vi "GUI_laptop v11i.vi"() -> ()   [LabVIEW 2019]
uses:
  <vilib>/Math Plots/3D Math Plots/3D Scatter/3D Scatter XCtrl/3D Scatter.xctl
  <vilib>/Platform/TimedLoop/XDataNode/timing_clust.ctl
  <vilib>/Platform/TimedLoop/XDataNode/nitl_modes.ctl
  <vilib>/Platform/TimedLoop/XDataNode/wakeup.ctl
  <vilib>/Analysis/_algsub.llb/Real Vector Norm.vi
  <vilib>/Instr/_visa.llb/VISA Configure Serial Port (Instr).vi
  <vilib>/Utility/file.llb/Write Delimited Spreadsheet (DBL).vi
  <vilib>/addons/System Identification/Data Preprocess.llb/SI Lowpass Filter (MISO Array).vi
  <vilib>/Math Plots/3D Math Plots/3D Scatter/3D Scatter Datatype/Public/Plot Helper (Vector).vi
  <vilib>/platform/TimedLoop/XDataNode/XDataNode.xnode
  <vilib>/Platform/TimedLoop/XDataNode/XDNodeRunTimeDep.lvlib
  <vilib>/Analysis/NI_AALPro.lvlib
  <vilib>/Math Plots/3D Math Plots/3D Scatter/3D Scatter Datatype/3D Scatter Datatype.lvclass
  <vilib>/addons/System Identification/NI_SysID.lvlib
panel:
  out "Period":i64
  out "Actual End [i-1]":i64
  out "Expected End [i-1]":i64
  out "Finished Late? [i-1] 2":bool
  in  "l3_init":dbl=2.0
  in  "Motion scale L3 outside rcm":dbl=2.0
  in  "L5 Deadzone":dbl
  in  "Sample rate":u32=500
  in  "Cutoff Frequency":dbl=10.0
  in  "Motion scale L1 L2":dbl=10.0
  in  "Motion scale L3":dbl=2.0
  in  "Save Path 4":path=path "C:/Users/jimmy/Documents/GitHub/Arduino-LabVIEW/zhantao/read_data_abs_filtered.csv"
  in  "Save Path 3":path=path "C:/Users/jimmy/Documents/GitHub/Arduino-LabVIEW/zhantao/read_data_abs_sending.csv"
  out "stimulus signals out":dbl[][](array[numeric]) format="%.2f"
  in  "L5 Offset":dbl
  in  "L5 Scale":dbl=1.0
  in  "Motion Scale L4":dbl=30.0
  out "spreadsheet string":string
  in  "Save Path 2":path=path "C:/Users/jimmy/Documents/GitHub/Arduino-LabVIEW/zhantao/read_data_delt.csv"
  out "send values":dbl[](array[numeric])
  out "Robot Feedback (l1 l2 l3 l4)":dbl[](array[numeric])
  in  "UDP Send":bool
  in  "UDP Recv":bool
  in  "L5 bound":dbl=1000.0
  in  "L4 bound (deg)":dbl=1000.0
  in  "L3 bound (mm)":dbl=1000.0
  in  "L2 bound (deg)":dbl=1000.0
  in  "L1 bound (deg)":dbl=1000.0
  in  "Joystick Type":dbl(ring)=1.0 items=["Rigid Joystick", "Free Joystick"]
  out "Finished Late? [i-1]":bool
  in  "Epsilon":dbl=0.2
  out "3D Scatter":refnum<class "3D Plot Datatype.lvclass">[](xcontrol)
  out "Random Point":dbl[](array[numeric])
  out "Virtual Cursor":dbl[](array[numeric])
  out "Iteration Duration":i64
  in  "Num of Points":i32=10
  in  "z bound":dbl=2.0
  in  "y bound":dbl=5.0
  in  "x bound":dbl=5.0
  in  "Stop":bool
  in  "Round Decimals":dbl=2.0 format="%#_15g"
  in  "Save Data":bool
  in  "Save Path":path=path "C:/Users/jimmy/Documents/GitHub/Arduino-LabVIEW/zhantao/read_data_abs.csv"
  in  "x speed":dbl=0.5
  in  "z speed":dbl=0.5
  in  "y speed":dbl=0.5
  out "error out":errorcluster
  in  "baud rate":u32=250000
  in  "VISA resource name":refnum<visa-resource-name>
  # "Joystick Selection"
  # "Plotting"
  # "Data Saving"
  # "Arduino Communication"
  # "Master Slave Communication"
  # "Parameters"
  # "TODO: add a lowpass filter for l5"
  # "TODO: fix the bounds; currently bounds are arbitrary"
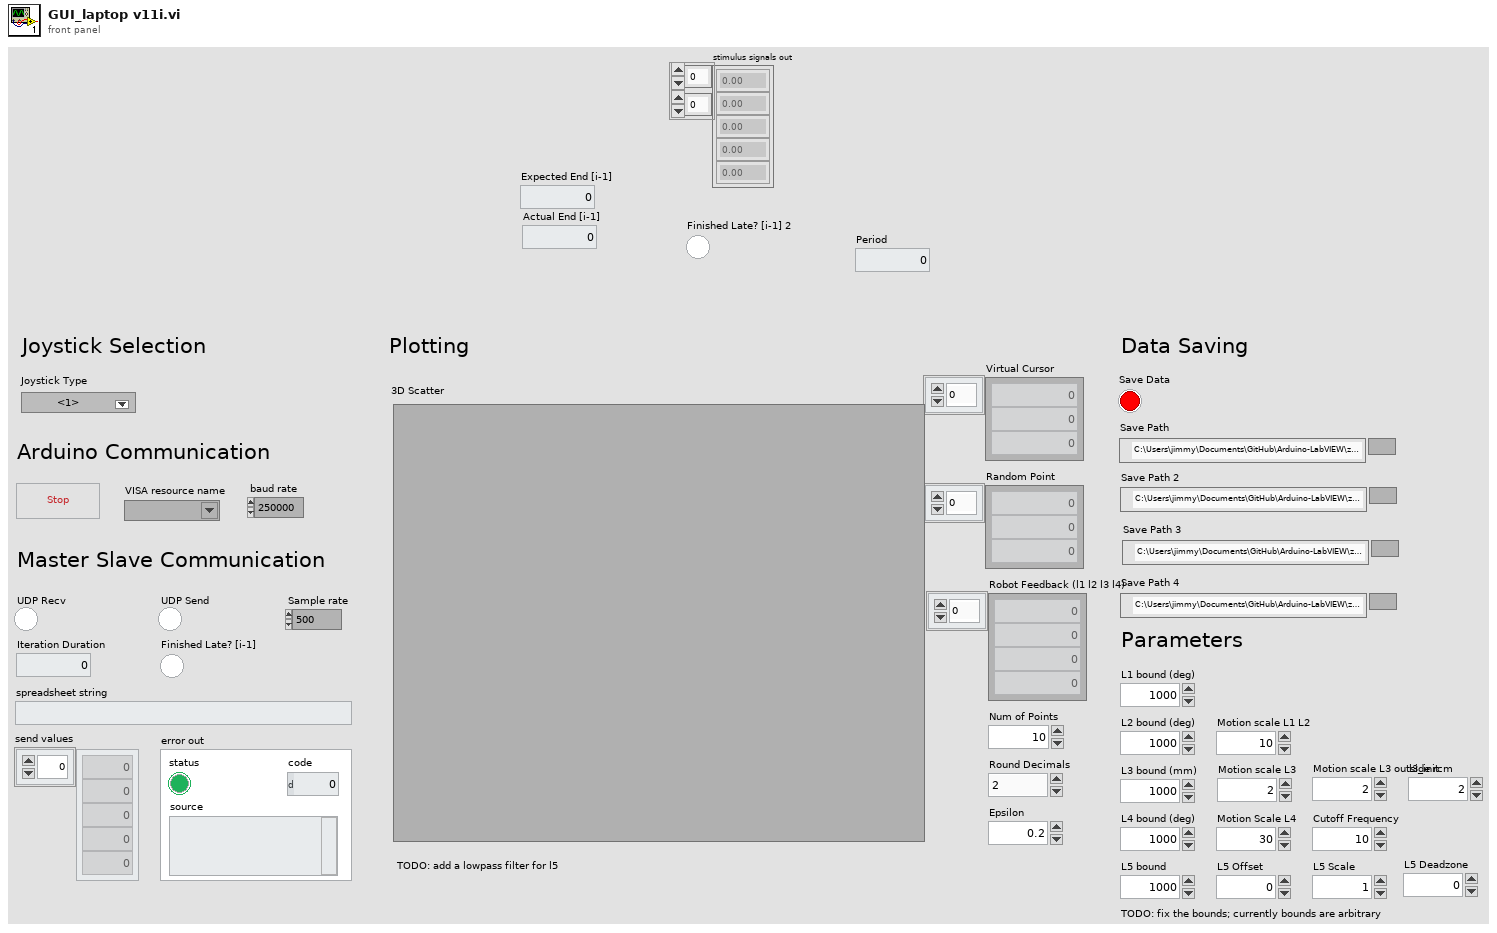
[diagram p1: front panel]
types:
  T1 = typedef "XDNodeRunTimeDep.lvlib/timing_clust.ctl" = cluster{"Expected End [f-1]":u64, "Actual End [f-1]":u64, "Finished Late? [f-1]":bool, "Expected End [i-1]":u64, "Actual End [i-1]":u64, "Finished Late? [i-1]":bool, "Expected Start [i]":u64, "Actual Start [i]":u64, "Expected Start [f]":u64, "Actual Start [f]":u64, "Source Name":string, "Structure Name":string, "Period":i64, "Deadline":i64, "Offset":i64, "Start":i64, "Priority":i32, "Timeout":i32, "Mode":T2, "Wakeup Reason":T3, "Error":errorcluster, "Source Type":string, "Secondary Source Type":string, "Global End Time":u64, "Global Start Time":u64, "Frame Duration":u64, "Iteration Duration":u64, "Assigned CPU":i32, "I/O Scan Engine Mode":u32}
  T2 = typedef "XDNodeRunTimeDep.lvlib/nitl_modes.ctl" = enum32{"No Change", "Process missed periods, maintain original phase", "Discard missed periods, maintain original phase", "Process missed periods, ignore original phase", "Discard missed periods, ignore original phase"}
  T3 = typedef "XDNodeRunTimeDep.lvlib/wakeup.ctl" = enum32{"Normal", "Aborted", "Asynchronous wakeup", "Timing source error", "Timed loop error", "Timeout"}
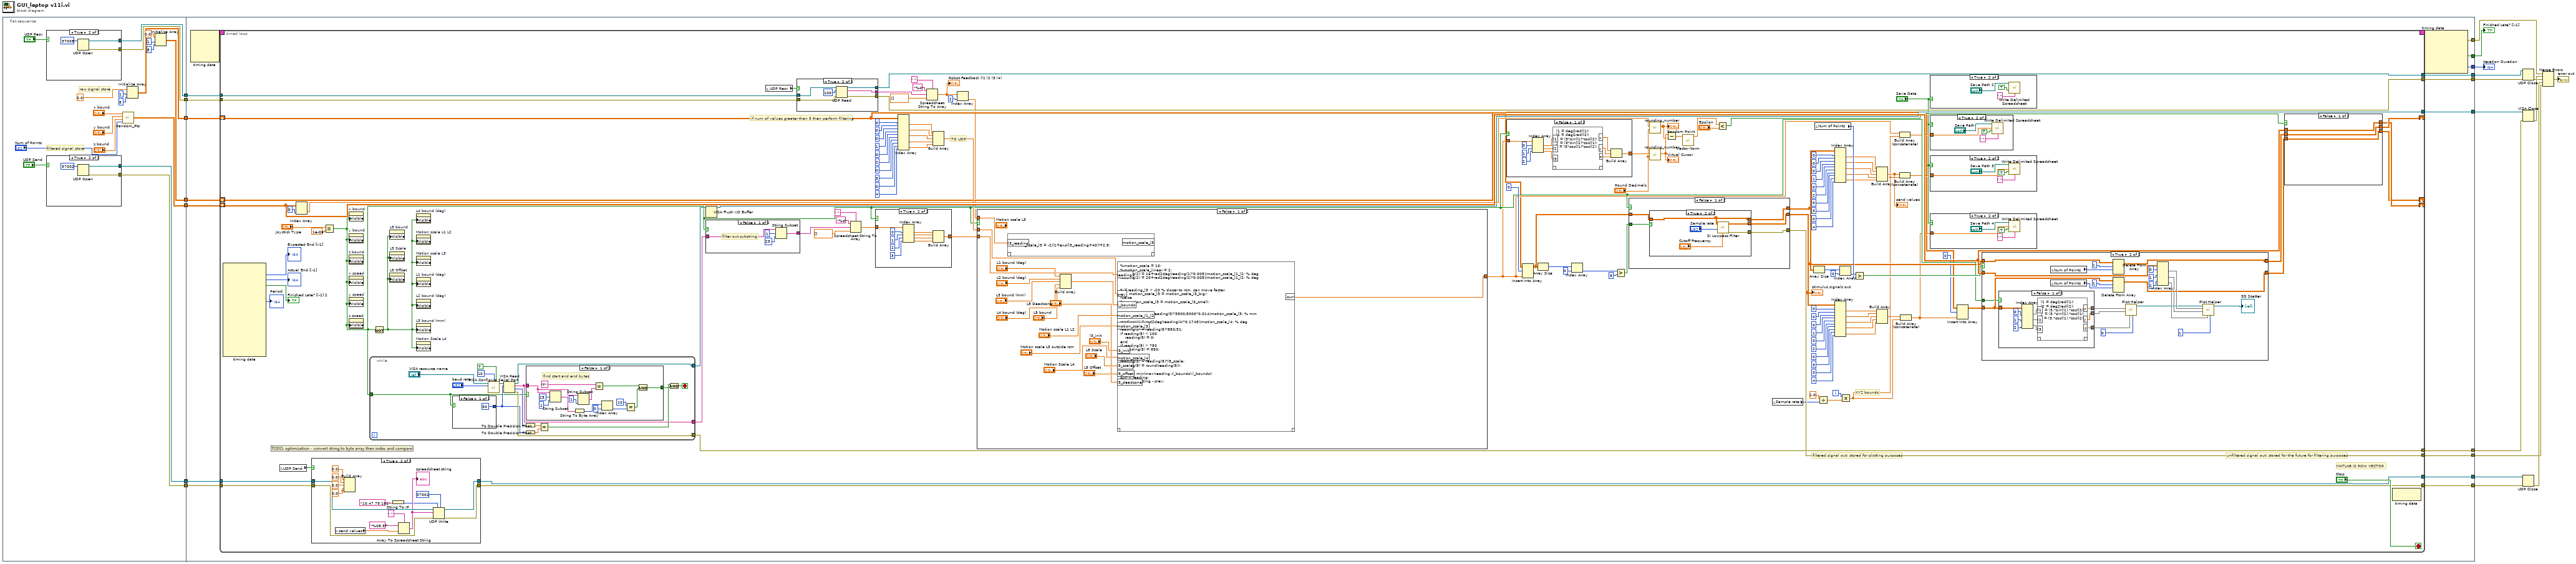
[diagram p0: block diagram]
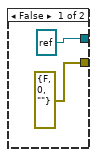
[diagram p2: hidden frame]
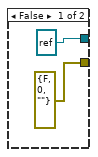
[diagram p3: hidden frame]
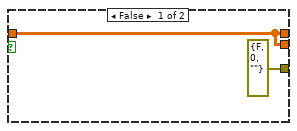
[diagram p6: hidden frame]
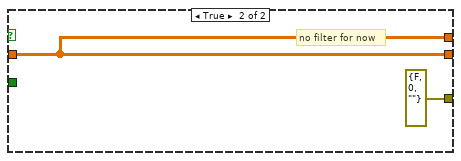
[diagram p7: hidden frame]
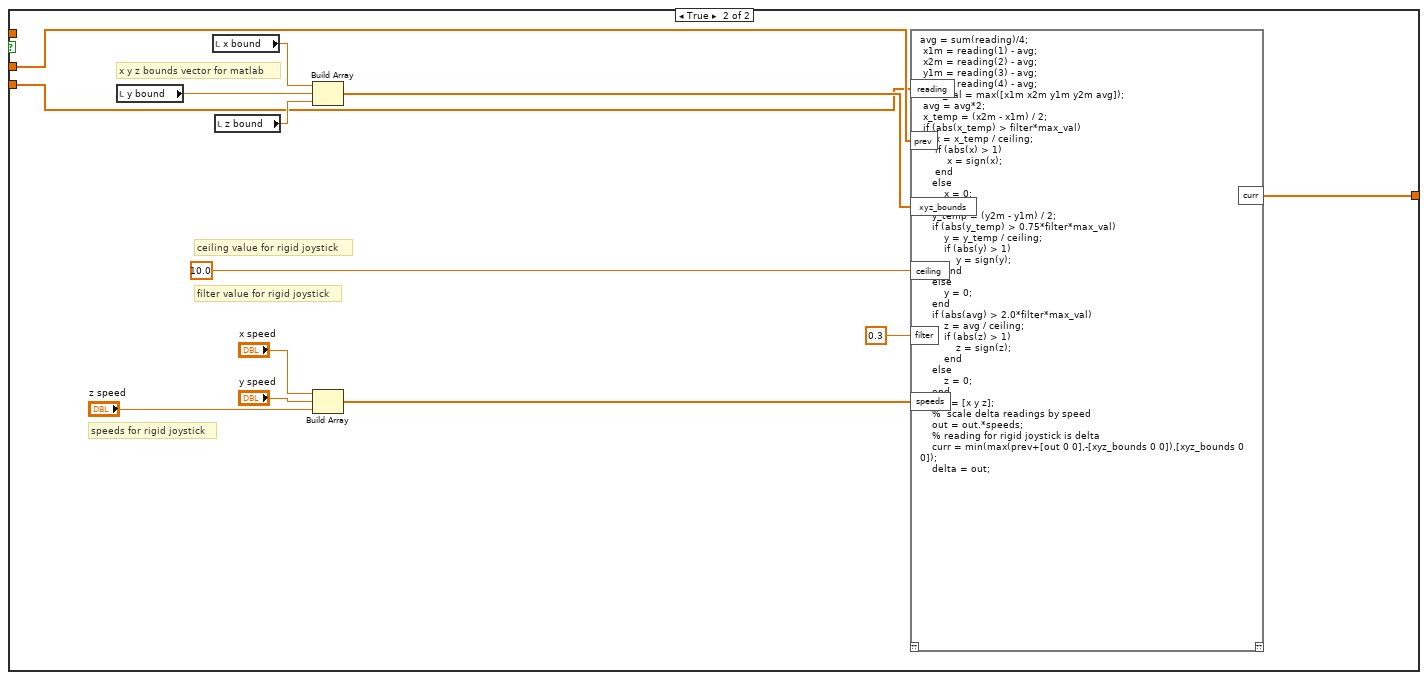
[diagram p8: hidden frame]
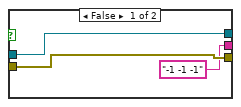
[diagram p11: hidden frame]
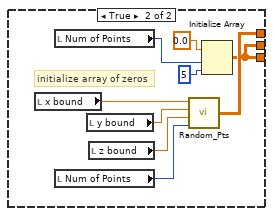
[diagram p13: hidden frame]
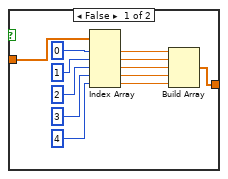
[diagram p15: hidden frame]
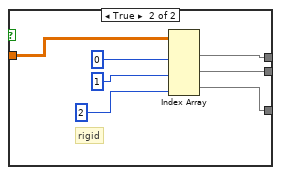
[diagram p18: hidden frame]
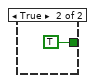
[diagram p19: hidden frame]
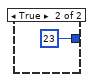
[diagram p20: hidden frame]
diagram:
  n1 = flat-sequence {
    tunnel: [w32] -> w18
    tunnel: [w36] -> w17
    tunnel: [w31] -> w16
    tunnel: [w30] -> w15
    tunnel: [w27] -> w14
    tunnel: [w26] -> w13
    tunnel: [w22] -> w2
    tunnel: [w67] -> w21
    tunnel: [w66] -> w20
    tunnel: [w64] -> w12
    tunnel: [w62] -> w19
    tunnel: w18 -> [w65]
    tunnel: w17 -> [w63]
    tunnel: w16 -> [w61]
    tunnel: w15 -> [w60]
    tunnel: w14 -> [w59]
    tunnel: w13 -> [w58]
    tunnel: [w57] -> w6
    tunnel: [w56] -> w11
    tunnel: [w55] -> w5
    tunnel: [w54] -> w4
    tunnel: [w53] -> w3
    tunnel: w2 -> [w52]
    tunnel: [w51] -> w1
    frame #0 {
      # "filtered signal store"
      # "raw signal store"
      n2 = case shown="True" "UDP Recv" {
        tunnel: [refnum<k16> refnum ("port") w49] -> w30
        tunnel: [errorcluster {"status"=FALSE, "code"=0, "source"=""} ("error out") w48] -> w27
        frame False {
        }
        frame True {
          n3 = UDP Open(11:u16 37008 ("port")) -> (port=w49:refnum<k16>, 0:w48:errorcluster)  [unwired: 4 in, 1 out]
        }
      }
      n4 = case shown="True" "UDP Send" {
        tunnel: [refnum<k16> refnum ("port") w44] -> w31
        tunnel: [errorcluster {"status"=FALSE, "code"=0, "source"=""} ("error out") w43] -> w26
        frame False {
        }
        frame True {
          n5 = UDP Open(11:u16 37002 ("port")) -> (port=w44:refnum<k16>, 0:w43:errorcluster)  [unwired: 4 in, 1 out]
        }
      }
      n6 = call "Random_Pts.vi"("Num of Points"="Num of Points", "z bound"="z bound", "y bound"="y bound", "x bound"="x bound") -> ("appended array"=w36:dbl[][])
      n7 = Initialize Array(0.0 ("element"), 1 ("dimension size"), 5 ("dimension size")) -> (w32:dbl[][])
      n8 = Initialize Array(0.0 ("element"), 1 ("dimension size"), 5 ("dimension size")) -> (w22:dbl[][])
    }
    frame #1 {
      n9 = node-c288() -> (w69:T1)  [unwired: 4 in]
      n10 = timed-loop {
        tunnel: [w141] -> w67
        tunnel: [w197] -> w66
        shift-right: [w196] -> _
        shift-left: w65 -> [w95]
        timing: w69 -> [_]
        timing-out: [_] -> w68
        shift-right: [w192] -> _
        shift-left: w63 -> [w193]
        tunnel: w61 -> [w155]
        tunnel: w60 -> [w154]
        tunnel: w59 -> [w152]
        tunnel: w58 -> [w151]
        tunnel: [w150] -> w57
        tunnel: [w149] -> w56
        tunnel: [w148] -> w55
        tunnel: [w147] -> w54
        tunnel: [w130] -> w53
        shift-right: [w86] -> _
        shift-left: w52 -> [w89]
        i -> [w84]
        stop <- "Stop" stop-if-true
        # "unfiltered signal out; stored for the future for filtering purposes"
        # "filtered signal out; stored for plotting purposes"
        # "XYZ bounds"
        # "if num of values greater than 5 then perform filtering"
        # "TO UDP"
        # "MATLAB IS ROW VECTOR"
        n11 = node-c288() -> (→"Expected End [i-1]":i64, →"Actual End [i-1]":i64, →"Finished Late? [i-1] 2":bool, →"Period":i64)  [unwired: 1 in, 12 out]
        n12 = local read "UDP Send"() -> (w79:bool)
        n13 = Index Array(array=w193, index (col)=0 ("index (row)")) -> (element=w164:dbl[])  [unwired: 1 in]
        n14 = case shown="True" w79 {
          tunnel: w155 -> [w254 w270]
          tunnel: w151 -> [w255 w266]
          tunnel: [w255 w262] -> w149
          tunnel: [w254 w261] -> w147
          frame False {
          }
          frame True {
            w260 = 0.0 ("element")
            n15 = local read "send values"() -> (w256:dbl[])
            n16 = Build Array(0.0 ("element"), 0.0 ("element"), 0.0 ("element"), w260, w260) -> ()  [unwired: 1 out]
            n17 = String To IP(1:"10.47.79.181" ("name")) -> (0:w264:u32)
            n18 = Array To Spreadsheet String(delimiter (Tab)=" ", array=w256, 3:"%08.3f" ("format string")) -> (spreadsheet string=w267:string)
            "spreadsheet string" <- w267
            n19 = UDP Write(address=w264, port or service name=u16 37001, connection ID=w270, data in=w267, 8:w266) -> (error out=w262:errorcluster, 3:w261:refnum<k16>)  [unwired: 1 in]
          }
        }
        n20 = Less Or Equal?(x="Joystick Type", y=1e-06) -> (x <= y?=w131:bool)
        n21 = property on="x bound" class="DigNum (strict)"("Visible"=w131) -> ()  [unwired: 2 in, 2 out]
        n22 = property on="y bound" class="DigNum (strict)"("Visible"=w131) -> ()  [unwired: 2 in, 2 out]
        n23 = property on="z bound" class="DigNum (strict)"("Visible"=w131) -> ()  [unwired: 2 in, 2 out]
        n24 = property on="x speed" class="DigNum (strict)"("Visible"=w131) -> ()  [unwired: 2 in, 2 out]
        n25 = property on="y speed" class="DigNum (strict)"("Visible"=w131) -> ()  [unwired: 2 in, 2 out]
        n26 = property on="z speed" class="DigNum (strict)"("Visible"=w131) -> ()  [unwired: 2 in, 2 out]
        n27 = while {
          tunnel: [w377] -> w166
          tunnel: [w390] -> w197
          tunnel: [w384] -> w142
          tunnel: w131 -> [w378]
          stop <- w380 stop-if-true
          n28 = case shown="False" w378 {
            tunnel: [30 u32 23 ("byte count")] -> w383
            frame False {
            }
            frame True {
            }
          }
          n29 = call-poly "VISA Configure Serial Port"("VISA resource name"="VISA resource name", "termination char\n(0xA = '\\n' = LF)"=u8 10 ("termination char\n(0xA = '\\n' = LF)"), "Enable Termination\nChar (T)"=TRUE ("Enable Termination\nChar (T)"), "baud rate (9600)"="baud rate") -> ("VISA resource name out"=w385:refnum<visa-resource-name>)  [unwired: 10 in, 1 out]
          n30 = VISA Read(VISA resource name=w385, byte count=w383) -> (VISA resource name out=w384:refnum<visa-resource-name>, read buffer=w377:string, return count=w392:u32, error out=w390:errorcluster)  [unwired: 1 in]
          n31 = To Double Precision Float(number=w392) -> (double precision float=w391:dbl)
          n32 = To Double Precision Float(number=w383) -> (double precision float=w382:dbl)
          n33 = case shown="False" w378 {
            tunnel: [w399 TRUE] -> w379
            tunnel: w377 -> [w402 _]
            frame False {
              # "find start and end bytes"
              n34 = String Subset(string=w402, offset (0)=29, length (rest)=1) -> (substring=w397:string)
              n35 = String To Byte Array(string=w397) -> (unsigned byte array=w396:u8[])
              n36 = String Subset(string=w402, length (rest)=1) -> (substring=w405:string)  [unwired: 1 in]
              n37 = Equal?(x="T", y=w405) -> (x = y?=w401:bool)
              n38 = Index Array(array=w396, index=0) -> (element=w394:u8)
              n39 = Equal?(x=10, y=w394) -> (x = y?=w400:bool)
              n40 = And(x=w401, y=w400) -> (x .and. y?=w399:bool)
            }
            frame True {
            }
          }
          n41 = Equal?(x=w391, y=w382) -> (x = y?=w381:bool)
          n42 = And(x=w381, y=w379) -> (x .and. y?=w380:bool)
        }
        n43 = Not(x=w131) -> (.not. x?=w93:bool)
        n44 = property on="L5 bound" class="DigNum (strict)"("Visible"=w93) -> ()  [unwired: 2 in, 2 out]
        n45 = property on="L5 Scale" class="DigNum (strict)"("Visible"=w93) -> ()  [unwired: 2 in, 2 out]
        n46 = property on="L5 Offset" class="DigNum (strict)"("Visible"=w93) -> ()  [unwired: 2 in, 2 out]
        n47 = property on="L4 bound (deg)" class="DigNum (strict)"("Visible"=w93) -> ()  [unwired: 2 in, 2 out]
        n48 = property on="Motion scale L1 L2" class="DigNum (strict)"("Visible"=w93) -> ()  [unwired: 2 in, 2 out]
        n49 = property on="Motion scale L3" class="DigNum (strict)"("Visible"=w93) -> ()  [unwired: 2 in, 2 out]
        n50 = property on="L1 bound (deg)" class="DigNum (strict)"("Visible"=w93) -> ()  [unwired: 2 in, 2 out]
        n51 = property on="L2 bound (deg)" class="DigNum (strict)"("Visible"=w93) -> ()  [unwired: 2 in, 2 out]
        n52 = property on="L3 bound (mm)" class="DigNum (strict)"("Visible"=w93) -> ()  [unwired: 2 in, 2 out]
        n53 = property on="Motion Scale L4" class="DigNum (strict)"("Visible"=w93) -> ()  [unwired: 2 in, 2 out]
        n54 = VISA Flush I/O Buffer(VISA resource name=w142) -> (VISA resource name out=w141:refnum<visa-resource-name>)  [unwired: 2 in, 1 out]
        n55 = case shown="False" w131 {
          tunnel: w166 -> [w299 w300]
          tunnel: [w296 w300] -> w165
          frame False {
            # "filter out substring"
            n56 = String Subset(string=w299, offset (0)=1, length (rest)=29) -> (substring=w296:string)
          }
          frame True {
          }
        }
        n57 = local read "UDP Recv"() -> (w153:bool)
        n58 = case shown="True" w153 {
          tunnel: w154 -> [w272 w279]
          tunnel: w152 -> [w273 w278]
          tunnel: [w273 w277] -> w150
          tunnel: [w272 w276] -> w148
          tunnel: ["-1 -1 -1" w274] -> w143
          frame False {
          }
          frame True {
            n59 = UDP Read(connection ID=w279, max size (548)=100, 8:w278) -> (data out=w274:string, error out=w277:errorcluster, 3:w276:refnum<k16>)  [unwired: 1 in, 2 out]
          }
        }
        n60 = Spreadsheet String To Array(delimiter (Tab)=",", format string="%d", spreadsheet string=w165, array type (2D Dbl)=dbl[] []) -> (array=w167:dbl[])
        n61 = case shown="True" w131 {
          tunnel: w167 -> [w301 w316]
          tunnel: [w306 w315] -> w139
          frame False {
            n62 = Index Array(array=w301, index #1=0 ("Plot ID"), index #2=1 ("Plot ID"), index #3=2 ("Plot ID"), index #4=3 ("Plot ID"), index #5=4 ("Plot ID")) -> (element #1=w309:dbl, element #2=w308:dbl, element #3=w307:dbl, element #4=w303:dbl, element #5=w302:dbl)
            n63 = Build Array(w309, w308, w307, w303, w302) -> (w306:dbl[])
          }
          frame True {
            n64 = Index Array(array=w316, index #1=0 ("Plot ID"), index #2=1 ("Plot ID"), index #3=2 ("Plot ID"), index #4=3 ("index")) -> (element #1=w319:dbl, element #2=w318:dbl, element #3=w317:dbl, element #4=w313:dbl)
            n65 = Build Array(w319, w318, w317, w313) -> (w315:dbl[])
          }
        }
        n66 = Index Array(array=w95, index (row) #1=0 ("disabled index (row)"), index (col) #1=0 ("disabled index (col)"), index (row) #2=0 ("disabled index (row)"), index (col) #2=1 ("disabled index (col)"), index (row) #3=0 ("disabled index (row)"), index (col) #3=2 ("disabled index (col)"), index (row) #4=0 ("disabled index (row)"), index (col) #4=3 ("disabled index (col)"), index (row) #5=0 ("disabled index (row)"), index (col) #5=4 ("disabled index (col)")) -> (element #1=w178:dbl, element #2=w177:dbl, element #3=w176:dbl, element #4=w169:dbl, element #5=w168:dbl)
        n67 = Spreadsheet String To Array(delimiter (Tab)=" ", format string="%d", spreadsheet string=w143, array type (2D Dbl)=dbl[] []) -> (array=w76:dbl[])
        "Robot Feedback (l1 l2 l3 l4)" <- w76
        n68 = Build Array(w178, w177, w176, w169, w168) -> (w140:dbl[])
        n69 = Index Array(array=w76, index=2) -> (element=w74:dbl)
        n70 = case shown="False" w131 {
          tunnel: w140 -> [w229 w240]
          tunnel: w139 -> [w230 w239]
          tunnel: [w228 w238] -> w114
          tunnel: w74 -> [w222 _]
          frame False {
            n71 = script code="motion_scale_l3 = -2/(1+exp(l3_reading+40))+2.5;"("l3_reading"=w222) -> ()  [unwired: 1 in, 2 out]
            n72 = Build Array("L1 bound (deg)", "L2 bound (deg)", "L3 bound (mm)", "L4 bound (deg)", "L5 bound") -> (w231:dbl[])
            n73 = script code="%motion_scale = 10;\n%motion_scale_linear = 2;\nreading(1) = 16+rad2deg(reading(1)*0.005)/motion_scale_l1_l2; % deg\nreading(2) = 20+rad2deg(reading(2)*0.005)/motion_scale_l1_l2; % deg\n\n\n%if reading_l3 > -20 % closer to rcm, can move faster;\n%    motion_scale_l3 = motion_scale_l3_big;;\n%else\n%   motion_scale_l3 = motion_scale_l3_small;\n%end\n\nreading(3) = -40-reading(3)*3500/3000*0.014/motion_scale_l3; % mm\n\nreading(4) = rad2deg(reading(4)*0.1745)/motion_scale_l4; % deg\n\nreading(5) = reading(5)*850/31;\nif reading(5) < 100\n    reading(5) = 0;\nend\nif reading(5) > 750\n    reading(5) = 850;\nend\n\nreading(5) = reading(5)*l5_scale;\nreading(5) = round(reading(5));\n\n%curr = min(max(reading,-l_bounds),l_bounds);\ncurr = reading;\ndelta = reading - prev;"("l_bounds"=w231, "motion_scale_l4"="Motion Scale L4", "reading"=w230, "prev"=w229, "l5_scale"="L5 Scale", "l5_offset"="L5 Offset", "motion_scale_l3"="Motion scale L3 outside rcm", "motion_scale_l1_l2"="Motion scale L1 L2", "l5_deadzone"="L5 Deadzone", "l3_init"="l3_init") -> ("curr"=w228:dbl[])  [unwired: 1 in, 1 out]
          }
          frame True {
            # "ceiling value for rigid joystick"
            # "filter value for rigid joystick"
            # "speeds for rigid joystick"
            # "x y z bounds vector for matlab"
            n74 = local read "y bound"() -> (w249:dbl)
            n75 = local read "x bound"() -> (w248:dbl)
            n76 = local read "z bound"() -> (w250:dbl)
            n77 = Build Array(w248, w249, w250) -> (w241:dbl[])
            n78 = Build Array("x speed", "y speed", "z speed") -> (w244:dbl[])
            n79 = script code="avg = sum(reading)/4;\n x1m = reading(1) - avg;\n x2m = reading(2) - avg;\n y1m = reading(3) - avg;\n y2m = reading(4) - avg;\n max_val = max([x1m x2m y1m y2m avg]);\n avg = avg*2;\n x_temp = (x2m - x1m) / 2;\n if (abs(x_temp) > filter*max_val)\n     x = x_temp / ceiling;\n     if (abs(x) > 1)\n         x = sign(x);\n     end\n    else\n        x = 0;\n    end\n    y_temp = (y2m - y1m) / 2;\n    if (abs(y_temp) > 0.75*filter*max_val)\n        y = y_temp / ceiling;\n        if (abs(y) > 1)\n            y = sign(y);\n        end\n    else\n        y = 0;\n    end\n    if (abs(avg) > 2.0*filter*max_val)\n        z = avg / ceiling;\n        if (abs(z) > 1)\n            z = sign(z);\n        end\n    else\n        z = 0;\n    end\n    out = [x y z];\n    %  scale delta readings by speed\n    out = out.*speeds;\n    % reading for rigid joystick is delta\n    curr = min(max(prev+[out 0 0],-[xyz_bounds 0 0]),[xyz_bounds 0 0]);\n    delta = out;"("xyz_bounds"=w241, "ceiling"=10.0 ("Real"), "filter"=0.3 ("Real"), "speeds"=w244, "reading"=w239, "prev"=w240) -> ("curr"=w238:dbl[])  [unwired: 1 in, 1 out]
          }
        }
        n80 = case shown="False" w131 {
          tunnel: [w327 w334] -> w194
          tunnel: w114 -> [w326 w334]
          frame False {
            n81 = Index Array(array=w326, index #1=0 ("Plot ID"), index #2=1 ("Plot ID"), index #3=2 ("Plot ID")) -> (element #1=w325:dbl, element #2=w324:dbl, element #3=w323:dbl)
            n82 = script code="l1 = deg2rad(l1);\nl2 = deg2rad(l2);\nx = l3*sin(l1)*cos(l2);\ny = l3*sin(l2)*cos(l1);\nz = l3*cos(l1)*cos(l2);"("l1"=w325, "l2"=w324, "l3"=w323) -> ("x"=w330:dbl, "y"=w329:dbl, "z"=w328:dbl)  [unwired: 1 in, 1 out]
            n83 = Build Array(w330, w329, w328) -> (w327:dbl[])
          }
          frame True {
          }
        }
        n84 = Insert Into Array(array=w95, index (row)=0, new element=w114) -> (w132:dbl[][])  [unwired: 1 in]
        n85 = Array Size(array=w132) -> (size(s)=w135:i32[])
        n86 = Index Array(array=w135, index=0) -> (element=w134:i32)
        n87 = Greater?(x=w134, y=5) -> (0:w80:bool)
        n88 = case shown="False" w131 {
          tunnel: w80 -> [w209 _]
          tunnel: w132 -> [w211 w219]
          tunnel: [w210 w219] -> w92
          tunnel: [w208 errorcluster {"status"=FALSE, "code"=0, "source"=""} ("error out")] -> w130
          tunnel: [w207 w219] -> w96
          frame False {
            n89 = case shown="True" w209 {
              tunnel: w211 -> [w212 w217]
              tunnel: [w212 w217] -> w210
              tunnel: [errorcluster {"status"=FALSE, "code"=0, "source"=""} ("error out") w218] -> w208
              tunnel: [w212 w216] -> w207
              frame False {
              }
              frame True {
                n90 = call-poly <vilib>:"SI Lowpass Filter.vi"("cutoff frequency"="Cutoff Frequency", "sampling rate (Hz)"="Sample rate", "stimulus signals in"=w217) -> ("error out"=w218:errorcluster, "stimulus signals out"=w216:dbl[][])  [unwired: 6 in, 1 out]
              }
            }
          }
          frame True {
            # "no filter for now"
          }
        }
        "stimulus signals out" <- w96
        n91 = call "rounding_number.vi"("power of ten"="Round Decimals", "Array"=w164) -> ("rounded"=w161:dbl[])  [unwired: 9 in]
        "Random Point" <- w161
        n92 = call "rounding_number.vi"("power of ten"="Round Decimals", "Array"=w194) -> ("rounded"=w162:dbl[])  [unwired: 9 in]
        "Virtual Cursor" <- w162
        n93 = Subtract(x=w162, y=w161) -> (x-y=w160:dbl[])
        n94 = call-poly <vilib>:"Vector Norm.vi"("Input Vector"=w160) -> ("norm"=w159:dbl)  [unwired: 9 in, 1 out]
        n95 = Less?(x=w159, y="Epsilon") -> (x < y?=w157:bool)
        n96 = local read "Sample rate"() -> (w81:u32)
        n97 = Array Size(array=w92) -> (size(s)=w138:i32[])
        n98 = local read "Num of Points"() -> (w180:i32)
        n99 = Divide(x=1.0, y=w81) -> (x/y=w82:dbl)
        n100 = Index Array(array=w92, index (row) #1=0 ("disabled index (col)"), index (col) #1=0 ("disabled index (row)"), index (row) #2=0 ("disabled index (col)"), index (col) #2=1 ("disabled index (row)"), index (row) #3=0 ("disabled index (col)"), index (col) #3=2 ("disabled index (row)"), index (row) #4=0 ("disabled index (col)"), index (col) #4=3 ("disabled index (row)"), index (row) #5=0 ("disabled index (col)"), index (col) #5=4 ("disabled index (col)")) -> (element #1=w119:dbl, element #2=w118:dbl, element #3=w117:dbl, element #4=w116:dbl, element #5=w115:dbl)
        n101 = Index Array(array=w96, index (row) #1=0 ("disabled index (col)"), index (col) #1=0 ("disabled index (row)"), index (row) #2=0 ("disabled index (col)"), index (col) #2=1 ("disabled index (row)"), index (row) #3=0 ("disabled index (col)"), index (col) #3=2 ("disabled index (row)"), index (row) #4=0 ("disabled index (col)"), index (col) #4=3 ("disabled index (row)"), index (row) #5=0 ("disabled index (col)"), index (col) #5=4 ("disabled index (col)")) -> (element #1=w102:dbl, element #2=w101:dbl, element #3=w100:dbl, element #4=w99:dbl, element #5=w98:dbl)
        n102 = Index Array(array=w138, index=0) -> (element=w181:i32)
        n103 = Multiply(x=w84, y=w82) -> (x*y=w85:dbl)
        n104 = Greater?(x=w181, y=w180) -> (0:w179:bool)
        n105 = Build Array(w119, w118, w117, w116, w115) -> (w77:dbl[])
        "send values" <- w77
        n106 = Build Array(w102, w101, w100, w99, w98) -> (w78:dbl[])
        n107 = Build Array (concatenate)(w114, w85) -> (w113:dbl[])
        n108 = Build Array (concatenate)(w77, w85) -> (w94:dbl[])
        n109 = Build Array (concatenate)(w78, w85) -> (w90:dbl[])
        n110 = case shown="True" "Save Data" {
          frame False {
          }
          frame True {
            n111 = call-poly <vilib>:"Write Delimited Spreadsheet.vi"("file path (dialog if empty)"="Save Path 2", "append to file? (new file:F)"=TRUE, "delimiter (\\t)"="," ("delimiter (\\t)")) -> ()  [unwired: 11 in, 2 out]
          }
        }
        n112 = case shown="True" "Save Data" {
          tunnel: w113 -> [_ w280]
          frame False {
          }
          frame True {
            n113 = call-poly <vilib>:"Write Delimited Spreadsheet.vi"("file path (dialog if empty)"="Save Path", "1D data"=w280, "append to file? (new file:F)"=TRUE, "delimiter (\\t)"="," ("delimiter (\\t)")) -> ()  [unwired: 10 in, 2 out]
          }
        }
        n114 = case shown="True" "Save Data" {
          tunnel: w94 -> [_ w203]
          frame False {
          }
          frame True {
            n115 = call-poly <vilib>:"Write Delimited Spreadsheet.vi"("file path (dialog if empty)"="Save Path 3", "1D data"=w203, "append to file? (new file:F)"=TRUE, "delimiter (\\t)"="," ("delimiter (\\t)")) -> ()  [unwired: 10 in, 2 out]
          }
        }
        n116 = case shown="True" "Save Data" {
          tunnel: w90 -> [_ w199]
          frame False {
          }
          frame True {
            n117 = call-poly <vilib>:"Write Delimited Spreadsheet.vi"("file path (dialog if empty)"="Save Path 4", "1D data"=w199, "append to file? (new file:F)"=TRUE, "delimiter (\\t)"="," ("delimiter (\\t)")) -> ()  [unwired: 10 in, 2 out]
          }
        }
        n118 = Insert Into Array(array=w89, index (row)=0, new element=w90) -> (w88:dbl[][])  [unwired: 1 in]
        n119 = case shown="True" w179 {
          tunnel: w92 -> [w336 w358]
          tunnel: [w336 w357] -> w195
          tunnel: w193 -> [w335 w356]
          tunnel: w131 -> [_ w341]
          tunnel: w88 -> [_ w338]
          tunnel: [w335 w337] -> w87
          frame False {
          }
          frame True {
            n120 = case shown="False" w341 {
              tunnel: w338 -> [w369 w373]
              tunnel: [w360 w372] -> w347
              tunnel: [w361 w371] -> w346
              tunnel: [w362 w370] -> w345
              frame False {
                n121 = Index Array(array=w369, index (col) #1=0 ("Plot ID"), index (col) #2=1 ("Plot ID"), index (col) #3=2 ("Plot ID")) -> (element #1=w365:dbl[], element #2=w364:dbl[], element #3=w363:dbl[])  [unwired: 3 in]
                n122 = script code="l1 = deg2rad(l1);\nl2 = deg2rad(l2);\nx = l3.*sin(l1).*cos(l2);\ny = l3.*sin(l2).*cos(l1);\nz = l3.*cos(l1).*cos(l2);"("l1"=w365, "l2"=w364, "l3"=w363) -> ("x"=w360:dbl[], "y"=w361:dbl[], "z"=w362:dbl[])  [unwired: 1 in, 1 out]
              }
              frame True {
                # "rigid"
                n123 = Index Array(array=w373, index (col) #1=0 ("disabled index (col)"), index (col) #2=1 ("index (col)"), index (col) #3=2 ("index (col)")) -> (element #1=w372:dbl[], element #2=w371:dbl[], element #3=w370:dbl[])  [unwired: 3 in]
              }
            }
            n124 = local read "Num of Points"() -> (w355:i32)
            n125 = local read "Num of Points"() -> (w340:i32)
            n126 = Delete From Array(array=w358, length=1, index (row)=w355) -> (array with subset deleted=w357:dbl[][])  [unwired: 1 in, 1 out]
            n127 = Delete From Array(array=w338, length=1, index (row)=w340) -> (array with subset deleted=w337:dbl[][])  [unwired: 1 in, 1 out]
            n128 = call-poly <vilib>:"Plot Helper.vi"("Plot ID"=0, "z vector"=w345, "y vector"=w346, "x vector"=w347) -> ("3D Plot lvclass Array out"=w349:refnum<class "3D Plot Datatype.lvclass">[])  [unwired: 2 in, 5 out]
            n129 = Index Array(array=w356, index (row) #1=0 ("index (row)"), index (row) #2=1 ("index (row)"), index (row) #3=2 ("index (row)")) -> (element #1=w353:dbl[], element #2=w352:dbl[], element #3=w351:dbl[])  [unwired: 3 in]
            n130 = call-poly <vilib>:"Plot Helper.vi"("Plot ID"=1, "z vector"=w351, "y vector"=w352, "x vector"=w353, "3D Plot lvclass Array in"=w349) -> ("3D Plot lvclass Array out"=→"3D Scatter":refnum<class "3D Plot Datatype.lvclass">[])  [unwired: 1 in, 5 out]
          }
        }
        n131 = case shown="False" w157 {
          tunnel: w193 -> [w286 _]
          tunnel: [w286 w291] -> w192
          tunnel: w195 -> [w285 _]
          tunnel: [w285 w287] -> w196
          tunnel: w87 -> [w284 _]
          tunnel: [w284 w287] -> w86
          frame False {
          }
          frame True {
            # "initialize array of zeros"
            n132 = local read "x bound"() -> (w295:dbl)
            n133 = local read "Num of Points"() -> (w289:i32)
            n134 = local read "Num of Points"() -> (w292:i32)
            n135 = local read "y bound"() -> (w294:dbl)
            n136 = local read "z bound"() -> (w293:dbl)
            n137 = call "Random_Pts.vi"("Num of Points"=w292, "z bound"=w293, "y bound"=w294, "x bound"=w295) -> ("appended array"=w291:dbl[][])
            n138 = Initialize Array(0.0 ("element"), w289, 5 ("dimension size")) -> (w287:dbl[][])
          }
        }
        n139 = node-c288() -> ()  [unwired: 1 in, 1 out]
      }
      n140 = node-c288(w68) -> (w64:errorcluster, w51:bool, w62:i64)  [unwired: 3 out]
    }
  }
  n141 = UDP Close(connection ID=w5, 8:w6) -> (error out=w9:errorcluster)  [unwired: 1 out]
  n142 = VISA Close(VISA resource name=w21, error in (no error)=w20) -> (error out=w10:errorcluster)
  n143 = UDP Close(connection ID=w4, 8:w11) -> (error out=w8:errorcluster)  [unwired: 1 out]
  n144 = Merge Errors(w12, w10, w9, w8, w3) -> (→"error out":errorcluster)
  "Iteration Duration" <- w19
  "Finished Late? [i-1]" <- w1
